vi "Sample_Scan_Pause.vi"(4 "waypoints path":path=path "C:/Users/ALS Measurement/Google Drive/LabVIEW/Thermionics Manipulator", 6 "Z tilt":dbl=10.0, 8 "Spacing [microns]":dbl=10.0, 9 "Long Side Speed [micron/s]":dbl=10.0, 10 "Scan Mode":T2=2 items=["Mode 1", "Mode 2", "Continuous 1", "Continuous 2"], 11 "VISA resource name":refnum<visa-resource-name>) -> (0 "velocity cluster":T1, 1 "Scan Time (hous:minutes:seconds)":string, 2 "Sample Scan Array":dbl[][](array[numeric]), 3 "VISA ressource out":refnum<visa-resource-name>, 5 "Number of Points":i32)   [LabVIEW 2018]
uses:
  Scan Mode.ctl
  ConversionAndInformation/Unit_Control.ctl
panel:
  in  "velocity cluster 2":T1
  out "Line Spacing (steps)":string="0"
  out "Scan Time (s)":dbl
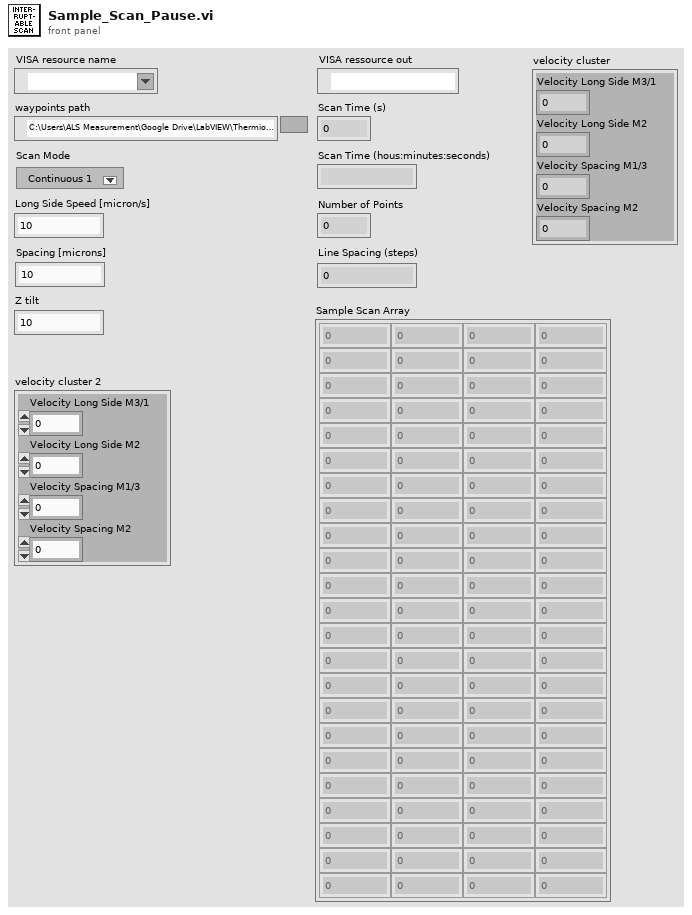
[diagram p1: front panel]
types:
  T1 = cluster{"Velocity Long Side M3/1":dbl, "Velocity Long Side M2":dbl, "Velocity Spacing M1/3":dbl, "Velocity Spacing M2":dbl}
  T2 = typedef "Scan Mode.ctl" = u16
  T3 = typedef "Unit_Control.ctl" = enum16{"Angle (Degrees)", "Rad", "Angle [TMC]", "Microsteps [TMC]", "Inches", "Nanometer", "Meter", "Centimeter", "Millimeter", "Micron"}
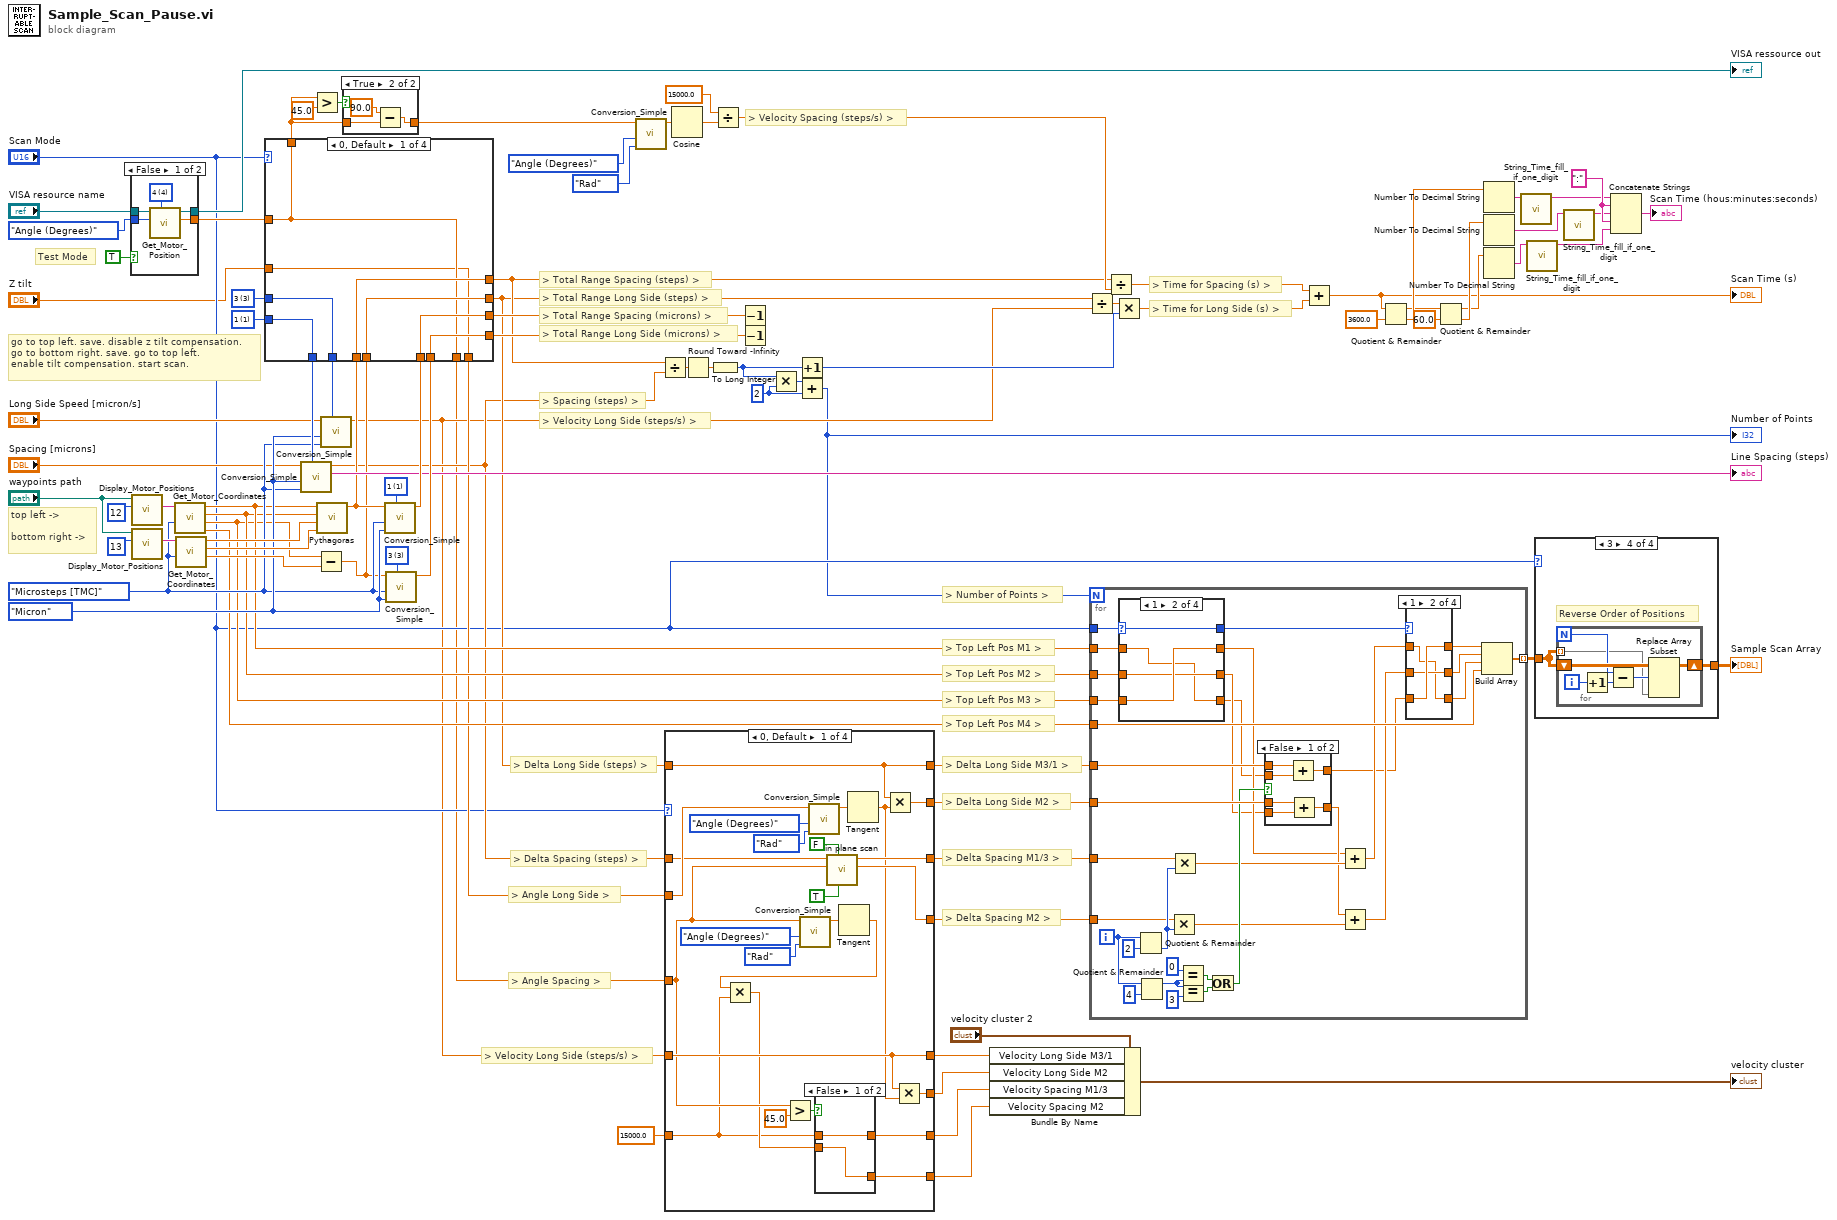
[diagram p0: block diagram]
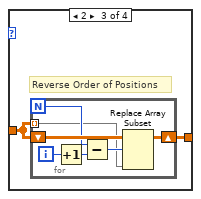
[diagram p4: hidden frame]
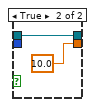
[diagram p5: hidden frame]
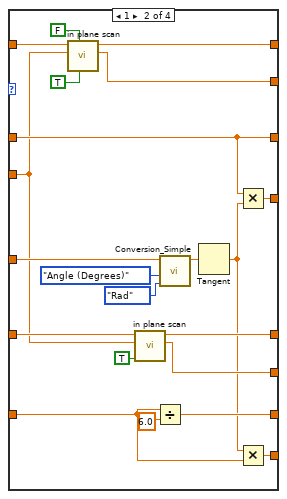
[diagram p7: hidden frame]
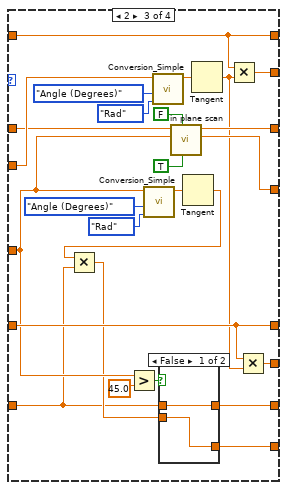
[diagram p8: hidden frame]
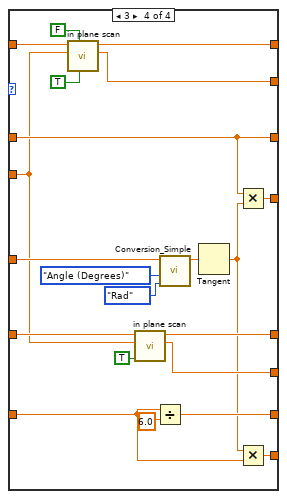
[diagram p10: hidden frame]
diagram:
  w51 = u16 3 items=["none", "1", "2", "3", "4", "all"] ("Motor")
  w52 = u16 1 items=["none", "1", "2", "3", "4", "all"] ("Motor")
  w57 = 2 ("y")
  w70 = ":"
  w55 = u16 1 items=["none", "1", "2", "3", "4", "all"] ("Motor")
  w82 = u16 3 items=["none", "1", "2", "3", "4", "all"] ("Motor")
  w50 = Unit_Control."Micron" ("Output Unit")
  w49 = Unit_Control."Microsteps [TMC]" ("Output Unit")
  # "> Velocity Long Side (steps/s) >"
  # "Test Mode"
  # "> Top Left Pos M4 >"
  # "go to top left. save. disable z tilt compensation.\ngo to bottom right. save. go to top left.\nenable tilt compensation. start scan."
  # "> Delta Spacing M2 >"
  # "> Delta Spacing M1/3 >"
  # "> Delta Long Side M2 >"
  # "> Delta Long Side M3/1 >"
  # "> Delta Spacing (steps) >"
  # "> Angle Spacing >"
  # "> Angle Long Side >"
  # "> Number of Points >"
  # "> Time for Long Side (s) >"
  # "> Time for Spacing (s) >"
  # "> Total Range Long Side (microns) >"
  # "> Total Range Long Side (steps) >"
  # "> Total Range Spacing (steps) >"
  # "> Total Range Spacing (microns) >"
  # "> Velocity Spacing (steps/s) >"
  # "> Spacing (steps) >"
  # "> Velocity Long Side (steps/s) >"
  # "> Delta Long Side (steps) >"
  # "> Top Left Pos M3 >"
  # "> Top Left Pos M2 >"
  # "> Top Left Pos M1 >"
  # "top left ->\n\nbottom right ->"
  n1 = case shown="False" TRUE {
    tunnel: "VISA resource name" -> [w95 w97]
    tunnel: Unit_Control."Angle (Degrees)" ("Output Unit") -> [w94 _]
    tunnel: [w92 10.0 ("Position")] -> w40
    tunnel: [w91 w97] -> w17
    frame False {
      w93 = u16 4 items=["none", "1", "2", "3", "4", "all"] ("Motor In")
      n2 = call "Get_Motor_Position.vi"("Motor In"=w93, "Output Unit"=w94, "VISA resource name"=w95) -> ("Position"=w92:dbl, "VISA ressource out"=w91:refnum<visa-resource-name>)  [unwired: 5 in, 2 out]
    }
    frame True {
    }
  }
  "VISA ressource out" <- w17
  n3 = call "Display_Motor_Positions.vi"("Waypoint Number"=12, "base path"="waypoints path") -> ("Loaded Positions"=w85:string)  [unwired: 8 in, 1 out]
  n4 = call "Display_Motor_Positions.vi"("Waypoint Number"=13, "base path"="waypoints path") -> ("Loaded Positions"=w84:string)  [unwired: 8 in, 1 out]
  n5 = call "Get_Motor_Coordinates.vi"("Output Unit"=w49, "string"=w85) -> ("Motor 4 Coordinate (deg)"=w27:dbl, "Motor 3 Coordinate"=w28:dbl, "Motor 2 Coordinate"=w29:dbl, "Motor 1 Coordinate"=w30:dbl)  [unwired: 6 in]
  n6 = call "Get_Motor_Coordinates.vi"("Output Unit"=w49, "string"=w84) -> ("Motor 3 Coordinate"=w90:dbl, "Motor 2 Coordinate"=w88:dbl, "Motor 1 Coordinate"=w89:dbl)  [unwired: 6 in, 1 out]
  n7 = Subtract(x=w28, y=w90) -> (x-y=w26:dbl)
  n8 = call "Pythagoras.vi"("Motor 2 Coordinate (bottom right)"=w88, "Motor 1 Coordinate (bottom right)"=w89, "Motor 2 Coordinate (top left)"=w29, "Motor 1 Coordinate (top left)"=w30) -> ("In Plain Distance"=w61:dbl)  [unwired: 7 in]
  n9 = call "Conversion_Simple.vi"("Motor"=w55, "Output Unit"=w50, "Input Unit"=w49, "Input"=w61) -> ("Output"=w81:dbl)  [unwired: 6 in, 1 out]
  n10 = call "Conversion_Simple.vi"("Motor"=w82, "Output Unit"=w50, "Input Unit"=w49, "Input"=w26) -> ("Output"=w80:dbl)  [unwired: 6 in, 1 out]
  n11 = case shown="0, Default" "Scan Mode" {
    tunnel: w81 -> [w105 w112 w121 w128]
    tunnel: [w105 w113 w121 w129] -> w47
    tunnel: w80 -> [w104 w113 w120 w129]
    tunnel: [w104 w112 w120 w128] -> w46
    tunnel: w61 -> [w100 w111 w116 w127]
    tunnel: w26 -> [w103 w108 w119 w124]
    tunnel: [w103 w111 w119 w127] -> w24
    tunnel: [w102 w110 w118 w126] -> w78
    tunnel: [w101 w109 w117 w125] -> w53
    tunnel: w52 -> [w102 w109 w118 w125]
    tunnel: w51 -> [w101 w110 w117 w126]
    tunnel: [w100 w108 w116 w124] -> w25
    tunnel: w40 -> [w99 w106 w115 w122]
    tunnel: "Z tilt" -> [w98 w107 w114 w123]
    tunnel: [w99 w107 w115 w123] -> w34
    tunnel: [w99 w107 w115 w123] -> w9
    tunnel: [w98 w106 w114 w122] -> w23
    frame 0, Default {
    }
    frame 1 {
    }
    frame 2 {
    }
    frame 3 {
    }
  }
  n12 = call "Conversion_Simple.vi"("Motor"=w78, "Output Unit"=w49, "Input Unit"=w50, "Input"="Spacing [microns]") -> (2:"Output"=→"Line Spacing (steps)":string, 3:"Output"=w22:dbl)  [unwired: 6 in]
  n13 = Greater?(x=w34, y=45.0) -> (0:w35:bool)
  n14 = call "Conversion_Simple.vi"("Motor"=w53, "Output Unit"=w49, "Input Unit"=w50, "Input"="Long Side Speed [micron/s]") -> ("Output"=w10:dbl)  [unwired: 6 in, 1 out]
  n15 = case shown="True" w35 {
    tunnel: w34 -> [w130 w133]
    tunnel: [w130 w131] -> w33
    frame False {
    }
    frame True {
      n16 = Subtract(x=90.0 ("y"), y=w133) -> (x-y=w131:dbl)
    }
  }
  n17 = call "Conversion_Simple.vi"("Output Unit"=Unit_Control."Rad" ("Input Unit"), "Input Unit"=Unit_Control."Angle (Degrees)", "Input"=w33) -> ("Output"=w38:dbl)  [unwired: 7 in, 1 out]
  n18 = Divide(x=w25, y=w22) -> (x/y=w83:dbl)
  n19 = case shown="0, Default" "Scan Mode" {
    tunnel: w24 -> [w153 w181 w203 w231]
    tunnel: w9 -> [w138 w172 w188 w222]
    tunnel: w23 -> [w152 w163 w202 w213]
    tunnel: w22 -> [w151 w175 w201 w225]
    tunnel: [w153 w180 w203 w230] -> w21
    tunnel: [w148 w179 w198 w229] -> w20
    tunnel: [w150 w175 w200 w225] -> w19
    tunnel: [w149 w174 w199 w224] -> w18
    tunnel: w10 -> [w147 w173 w197 w223]
    tunnel: 15000.0 -> [w134 w165 w184 w215]
    tunnel: [w147 w170 w197 w220] -> w6
    tunnel: [w145 w169 w195 w219] -> w5
    tunnel: [w142 w168 w192 w218] -> w4
    tunnel: [w141 w166 w191 w216] -> w3
    frame 0, Default {
      n20 = Greater?(x=w138, y=45.0) -> (0:w143:bool)
      n21 = call "Conversion_Simple.vi"("Output Unit"=Unit_Control."Rad", "Input Unit"=Unit_Control."Angle (Degrees)", "Input"=w138) -> ("Output"=w139:dbl)  [unwired: 7 in, 1 out]
      n22 = call "Conversion_Simple.vi"("Output Unit"=Unit_Control."Rad", "Input Unit"=Unit_Control."Angle (Degrees)", "Input"=w152) -> ("Output"=w155:dbl)  [unwired: 7 in, 1 out]
      n23 = call "in plane scan.vi"("invert y"=TRUE, "invert x"=FALSE, "angle (degrees)"=w138, "v total"=w151) -> ("v_y"=w149:dbl, "v_x"=w150:dbl)  [unwired: 2 in, 4 out]
      n24 = Tangent(1:w139) -> (0:w135:dbl)
      n25 = Multiply(x=w135, y=w134) -> (x*y=w137:dbl)
      n26 = case shown="False" w143 {
        tunnel: w134 -> [w160 w162]
        tunnel: [w160 w161] -> w142
        tunnel: [w159 w162] -> w141
        tunnel: w137 -> [w159 w161]
        frame False {
        }
        frame True {
        }
      }
      n27 = Tangent(1:w155) -> (0:w146:dbl)
      n28 = Multiply(x=w153, y=w146) -> (x*y=w148:dbl)
      n29 = Multiply(x=w147, y=w146) -> (x*y=w145:dbl)
    }
    frame 1 {
      n30 = call "in plane scan.vi"("invert y"=TRUE, "invert x"=FALSE, "angle (degrees)"=w163, "v total"=w181) -> ("v_y"=w179:dbl, "v_x"=w180:dbl)  [unwired: 2 in, 4 out]
      n31 = call "in plane scan.vi"("abs(x,y)"=TRUE ("invert y"), "angle (degrees)"=w163, "v total"=w173) -> ("v_y"=w169:dbl, "v_x"=w170:dbl)  [unwired: 3 in, 4 out]
      n32 = Divide(x=w165, y=6.0) -> (x/y=w168:dbl)
      n33 = call "Conversion_Simple.vi"("Output Unit"=Unit_Control."Rad", "Input Unit"=Unit_Control."Angle (Degrees)", "Input"=w172) -> ("Output"=w177:dbl)  [unwired: 7 in, 1 out]
      n34 = Tangent(1:w177) -> (0:w164:dbl)
      n35 = Multiply(x=w175, y=w164) -> (x*y=w174:dbl)
      n36 = Multiply(x=w164, y=w165) -> (x*y=w166:dbl)
    }
    frame 2 {
      n37 = Greater?(x=w188, y=45.0) -> (0:w193:bool)
      n38 = call "Conversion_Simple.vi"("Output Unit"=Unit_Control."Rad", "Input Unit"=Unit_Control."Angle (Degrees)", "Input"=w188) -> ("Output"=w189:dbl)  [unwired: 7 in, 1 out]
      n39 = call "Conversion_Simple.vi"("Output Unit"=Unit_Control."Rad", "Input Unit"=Unit_Control."Angle (Degrees)", "Input"=w202) -> ("Output"=w205:dbl)  [unwired: 7 in, 1 out]
      n40 = call "in plane scan.vi"("invert y"=TRUE, "invert x"=FALSE, "angle (degrees)"=w188, "v total"=w201) -> ("v_y"=w199:dbl, "v_x"=w200:dbl)  [unwired: 2 in, 4 out]
      n41 = Tangent(1:w189) -> (0:w185:dbl)
      n42 = Multiply(x=w185, y=w184) -> (x*y=w187:dbl)
      n43 = case shown="False" w193 {
        tunnel: w184 -> [w210 w212]
        tunnel: [w210 w211] -> w192
        tunnel: [w209 w212] -> w191
        tunnel: w187 -> [w209 w211]
        frame False {
        }
        frame True {
        }
      }
      n44 = Tangent(1:w205) -> (0:w196:dbl)
      n45 = Multiply(x=w203, y=w196) -> (x*y=w198:dbl)
      n46 = Multiply(x=w197, y=w196) -> (x*y=w195:dbl)
    }
    frame 3 {
      n47 = call "in plane scan.vi"("invert y"=TRUE, "invert x"=FALSE, "angle (degrees)"=w213, "v total"=w231) -> ("v_y"=w229:dbl, "v_x"=w230:dbl)  [unwired: 2 in, 4 out]
      n48 = call "in plane scan.vi"("abs(x,y)"=TRUE ("invert y"), "angle (degrees)"=w213, "v total"=w223) -> ("v_y"=w219:dbl, "v_x"=w220:dbl)  [unwired: 3 in, 4 out]
      n49 = Divide(x=w215, y=6.0) -> (x/y=w218:dbl)
      n50 = call "Conversion_Simple.vi"("Output Unit"=Unit_Control."Rad", "Input Unit"=Unit_Control."Angle (Degrees)", "Input"=w222) -> ("Output"=w227:dbl)  [unwired: 7 in, 1 out]
      n51 = Tangent(1:w227) -> (0:w214:dbl)
      n52 = Multiply(x=w225, y=w214) -> (x*y=w224:dbl)
      n53 = Multiply(x=w214, y=w215) -> (x*y=w216:dbl)
    }
  }
  n54 = Cosine(x=w38) -> (cos(x)=w32:dbl)
  n55 = Round Toward -Infinity(1:w83) -> (0:w79:dbl)
  n56 = To Long Integer(number=w79) -> (32bit integer=w56:i32)
  n57 = Divide(x=15000.0, y=w32) -> (x/y=w31:dbl)
  n58 = Decrement(x=w47) -> ()  [unwired: 1 out]
  n59 = Decrement(x=w46) -> ()  [unwired: 1 out]
  n60 = Multiply(x=w56, y=w57) -> (x*y=w58:i32)
  n61 = Increment(x=w56) -> (x+1=w44:i32)
  n62 = Add(x=w58, y=w57) -> (x+y=w1:i32)
  "Number of Points" <- w1
  n63 = Bundle By Name(cluster="velocity cluster 2", "Velocity Long Side M3/1"=w6, "Velocity Long Side M2"=w5, "Velocity Spacing M1/3"=w4, "Velocity Spacing M2"=w3) -> (→"velocity cluster":T1)
  n64 = Divide(x=w24, y=w10) -> (x/y=w45:dbl)
  n65 = for {
    N: w1 -> [_]
    tunnel: w30 -> [w247]
    tunnel: w29 -> [w246]
    tunnel: w28 -> [w242]
    tunnel: [w259] -> w14 mode=indexing
    tunnel: w27 -> [w245]
    tunnel: w21 -> [w254]
    tunnel: w20 -> [w253]
    tunnel: w19 -> [w256]
    tunnel: w18 -> [w255]
    tunnel: "Scan Mode" -> [w248]
    i -> [w264]
    n66 = case shown="1" w248 {
      selector: w248 -> [w279 w283 w287 w291]
      tunnel: w247 -> [w282 w284 w290 w292]
      tunnel: w246 -> [w281 w285 w289 w293]
      tunnel: w242 -> [w280 w286 w288 w294]
      tunnel: [w282 w286 w290 w294] -> w244
      tunnel: [w281 w285 w289 w293] -> w243
      tunnel: [w280 w284 w288 w292] -> w241
      tunnel: [w279 w283 w287 w291] -> w240
      frame 0, Default {
      }
      frame 1 {
      }
      frame 2 {
      }
      frame 3 {
      }
    }
    n67 = Quotient & Remainder(x=w264, y=2) -> (floor(x/y)=w257:i32)  [unwired: 1 out]
    n68 = Quotient & Remainder(x=w264, y=4) -> (x-y*floor(x/y)=w258:i32)  [unwired: 1 out]
    n69 = Multiply(x=w255, y=w257) -> (x*y=w251:dbl)
    n70 = Multiply(x=w256, y=w257) -> (x*y=w250:dbl)
    n71 = Equal?(x=0 ("y"), y=w258) -> (x = y?=w261:bool)
    n72 = Equal?(x=w258, y=3) -> (x = y?=w260:bool)
    n73 = Or(x=w261, y=w260) -> (x .or. y?=w252:bool)
    n74 = case shown="False" w252 {
      tunnel: w253 -> [w299 _]
      tunnel: w254 -> [w300 _]
      tunnel: w243 -> [w298 w301]
      tunnel: w241 -> [w297 w302]
      tunnel: [w296 w302] -> w237
      tunnel: [w295 w301] -> w249
      frame False {
        n75 = Add(x=w300, y=w297) -> (x+y=w296:dbl)
        n76 = Add(x=w299, y=w298) -> (x+y=w295:dbl)
      }
      frame True {
      }
    }
    n77 = Add(x=w244, y=w250) -> (x+y=w239:dbl)
    n78 = Add(x=w249, y=w251) -> (x+y=w238:dbl)
    n79 = case shown="1" w240 {
      tunnel: w239 -> [w269 w270 w275 w276]
      tunnel: w238 -> [w268 w271 w274 w277]
      tunnel: w237 -> [w267 w272 w273 w278]
      tunnel: [w269 w272 w275 w278] -> w236
      tunnel: [w268 w271 w274 w277] -> w235
      tunnel: [w267 w270 w273 w276] -> w234
      frame 0, Default {
      }
      frame 1 {
      }
      frame 2 {
      }
      frame 3 {
      }
    }
    n80 = Build Array(w236, w235, w234, w245) -> (w259:dbl[])
  }
  n81 = Divide(x=w25, y=w31) -> (x/y=w42:dbl)
  n82 = Multiply(x=w45, y=w44) -> (x*y=w43:dbl)
  n83 = Add(x=w42, y=w43) -> (x+y=w41:dbl)
  "Scan Time (s)" <- w41
  n84 = Quotient & Remainder(x=w41, y=3600.0) -> (x-y*floor(x/y)=w73:dbl, floor(x/y)=w75:dbl)
  n85 = Quotient & Remainder(x=w73, y=60.0) -> (x-y*floor(x/y)=w71:dbl, floor(x/y)=w72:dbl)
  n86 = Number To Decimal String(number=w75) -> (decimal integer string=w68:string)  [unwired: 1 in]
  n87 = Number To Decimal String(number=w72) -> (decimal integer string=w66:string)  [unwired: 1 in]
  n88 = Number To Decimal String(number=w71) -> (decimal integer string=w64:string)  [unwired: 1 in]
  n89 = call "String_Time_fill_if_one_digit.vi"("String"=w68) -> ("String 2"=w67:string)  [unwired: 10 in]
  n90 = call "String_Time_fill_if_one_digit.vi"("String"=w64) -> ("String 2"=w63:string)  [unwired: 10 in]
  n91 = case shown="3" "Scan Mode" {
    tunnel: w14 -> [w303 w304 w306 w315]
    tunnel: [w303 w304 w305 w314] -> w13
    frame 0, Default {
    }
    frame 1 {
    }
    frame 2 {
      # "Reverse Order of Positions"
      n92 = for {
        N -> [w311]
        tunnel: w306 -> [w309] mode=indexing
        shift-right: [w312] -> w305
        shift-left: w306 -> [w313]
        i -> [w308]
        n93 = Increment(x=w308) -> (x+1=w307:i32)
        n94 = Subtract(x=w311, y=w307) -> (x-y=w310:i32)
        n95 = Replace Array Subset(array=w313, new element=w309, index (row)=w310) -> (w312:dbl[][])  [unwired: 1 in]
      }
    }
    frame 3 {
      # "Reverse Order of Positions"
      n96 = for {
        N -> [w320]
        tunnel: w315 -> [w318] mode=indexing
        shift-right: [w321] -> w314
        shift-left: w315 -> [w322]
        i -> [w317]
        n97 = Increment(x=w317) -> (x+1=w316:i32)
        n98 = Subtract(x=w320, y=w316) -> (x-y=w319:i32)
        n99 = Replace Array Subset(array=w322, new element=w318, index (row)=w319) -> (w321:dbl[][])  [unwired: 1 in]
      }
    }
  }
  "Sample Scan Array" <- w13
  n100 = call "String_Time_fill_if_one_digit.vi"("String"=w66) -> ("String 2"=w65:string)  [unwired: 10 in]
  n101 = Concatenate Strings(w67, w70, w65, w70, w63) -> (→"Scan Time (hous:minutes:seconds)":string)
